vi "Teleop.vi"(10 "Match Info":T1={"Autonomous Elapsed Seconds"=0.0, "TeleOp Elapsed Seconds"=0.0, "Disabled Elapsed Seconds"=0.0, "Visited Autonomous"=FALSE, "Visited TeleOp"=FALSE, "Visited Disabled"=FALSE, "Autonomous Settings"={"Autonomous Style"=enum."Independent", "VI Refnum"=refnum}}, 11 "Call Context":T2) -> ()   [LabVIEW 2019]
doc: "This VI is called for each TeleOp packet received from the DS where the robot is not disabled. It is often used to read from the joysticks and update I/O or to update setpoints for timed control loops. It should complete and return within 20 milliseconds or it may miss DS packets."
uses:
  <vilib>/Rock Robotics/WPI/DriverStation/WPI_DriverStationDerivedRobotMode.ctl
  <vilib>/Rock Robotics/WPI/DriverStation/WPI_DriverStationMatch Info.ctl
  <vilib>/Rock Robotics/WPI/Solenoid/WPI_SolenoidValue.ctl
  <vilib>/Rock Robotics/WPI/Utilities/WPI_GetSetVariantRefNum.vi
  <vilib>/Rock Robotics/Network Tables/NT Write Boolean Array.vi
  <vilib>/Rock Robotics/Network Tables/NT Write Numeric Array.vi
  <vilib>/Rock Robotics/Network Tables/NT Read Boolean.vi
  <vilib>/Rock Robotics/Network Tables/NT Read Number.vi
  <vilib>/Rock Robotics/WPI/Solenoid/WPI_SolenoidSetEnum.vi
panel:
  in  "Auto speed switch":dbl=0.75
  out "Buttons":bool[](array[boolean])
  out "Axes":dbl[](array[numeric])
  out "Sample Slider 0":dbl(slide) scale=0.0..5.0
  out "Sample Boolean 1":bool
  # "REMEMBER BETWEEN 0 AND 1"
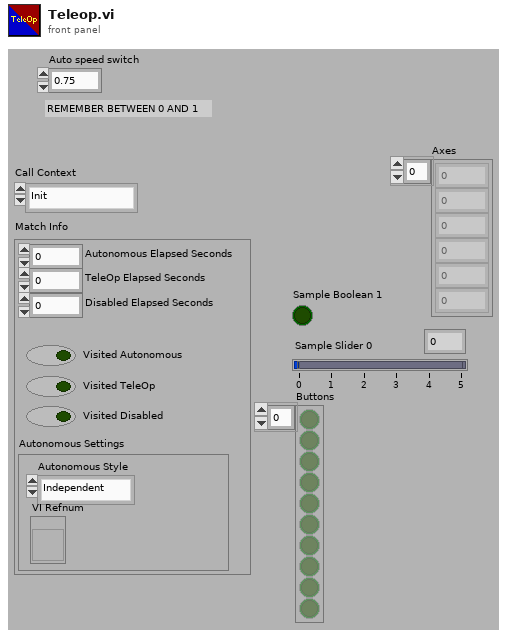
[diagram p1: front panel]
types:
  T1 = typedef "WPI_DriverStationMatch Info.ctl" = cluster{"Autonomous Elapsed Seconds":dbl, "TeleOp Elapsed Seconds":dbl, "Disabled Elapsed Seconds":dbl, "Visited Autonomous":bool, "Visited TeleOp":bool, "Visited Disabled":bool, "Autonomous Settings":cluster{"Autonomous Style":enum16{"Iterative", "Independent"}, "VI Refnum":refnum<vi>}}
  T2 = typedef "WPI_DriverStationDerivedRobotMode.ctl" = enum16{"Init", "Execute", "Stop"}
  T3 = typedef "WPI_JoystickDevRef.ctl" = cluster{"Device":T4}
  T4 = typedef "WPI_JoystickDeviceEnum.ctl" = enum16{"USB 0", "USB 1", "USB 2", "USB 3", "USB 4", "USB 5"}
  T5 = typedef "WPI_SolenoidValue.ctl" = enum16{"Off", "On", "Forward", "Reverse"}
  T6 = typedef "WPI_SolenoidDevRef.ctl" = cluster{"DevStatus":errorcluster, "Pneumatics Control Module":u8, "Forward Solenoid Channel":T7, "Reverse Solenoid Channel":T7}
  T7 = typedef "WPI_SolenoidChannel.ctl" = enum8{"Solenoid 0", "Solenoid 1", "Solenoid 2", "Solenoid 3", "Solenoid 4", "Solenoid 5", "Solenoid 6", "Solenoid 7", "Invalid"}
  T8 = typedef "WPI_RobotDriveDevRef.ctl" = cluster{"DevStatus":errorcluster, "Motors[]":T9[], "Square Inputs":bool, "Max Output":dbl}
  T9 = typedef "WPI_MotorControlDeviceRef.ctl" = cluster{"DeviceStatus":errorcluster, "Type":T10, "PWM":cluster{"PWM Channel":T11, "DeadBand":T12}, "CAN":cluster{"Device Number":u8, "SetOutput VI Ref":variant, "GetOutput VI Ref":variant, "Enable VI Ref":variant, "Disable VI Ref":variant, "Data":variant}, "Invert":bool, "DIO PWM":cluster{"PWM \"Enable\" Channel":T11, "DIOChannel":T13, "PWM Rate":dbl}}
  T10 = typedef "WPI_MotorControlType.ctl" = enum16{"PWM", "CAN", "DIO PWM"}
  T11 = typedef "FPGA_DIOPWMChannel.ctl" = enum8{"PWM 0", "PWM 1", "PWM 2", "PWM 3", "PWM 4", "PWM 5", "PWM 6", "PWM 7", "PWM 8", "PWM 9", "PWM MXP 0", "PWM MXP 1", "PWM MXP 2", "PWM MXP 3", "PWM MXP 4", "PWM MXP 5", "PWM MXP 6", "PWM MXP 7", "PWM MXP 8", "PWM MXP 9", "Invalid"}
  T12 = typedef "WPI_PWMDeadband.ctl" = cluster{"Name":string, "maxPositivePwm":i32, "minPositivePwm":i32, "centerPwm":i32, "maxNegativePwm":i32, "minNegativePwm":i32, "angularRange":u16}
  T13 = typedef "FPGA_DIOChannel.ctl" = enum8{"DIO 0", "DIO 1", "DIO 2", "DIO 3", "DIO 4", "DIO 5", "DIO 6", "DIO 7", "DIO 8", "DIO 9", "DIO MXP 0", "DIO MXP 1", "DIO MXP 2", "DIO MXP 3", "DIO MXP 4", "DIO MXP 5", "DIO MXP 6", "DIO MXP 7", "DIO MXP 8", "DIO MXP 9", "DIO MXP 10", "DIO MXP 11", "DIO MXP 12", "DIO MXP 13", "DIO MXP 14", "DIO MXP 15", "SPI Port CS1", "SPI Port CS2", "SPI Port CS3", "SPI Port MISO", "SPI Port MOSI", "Invalid"}
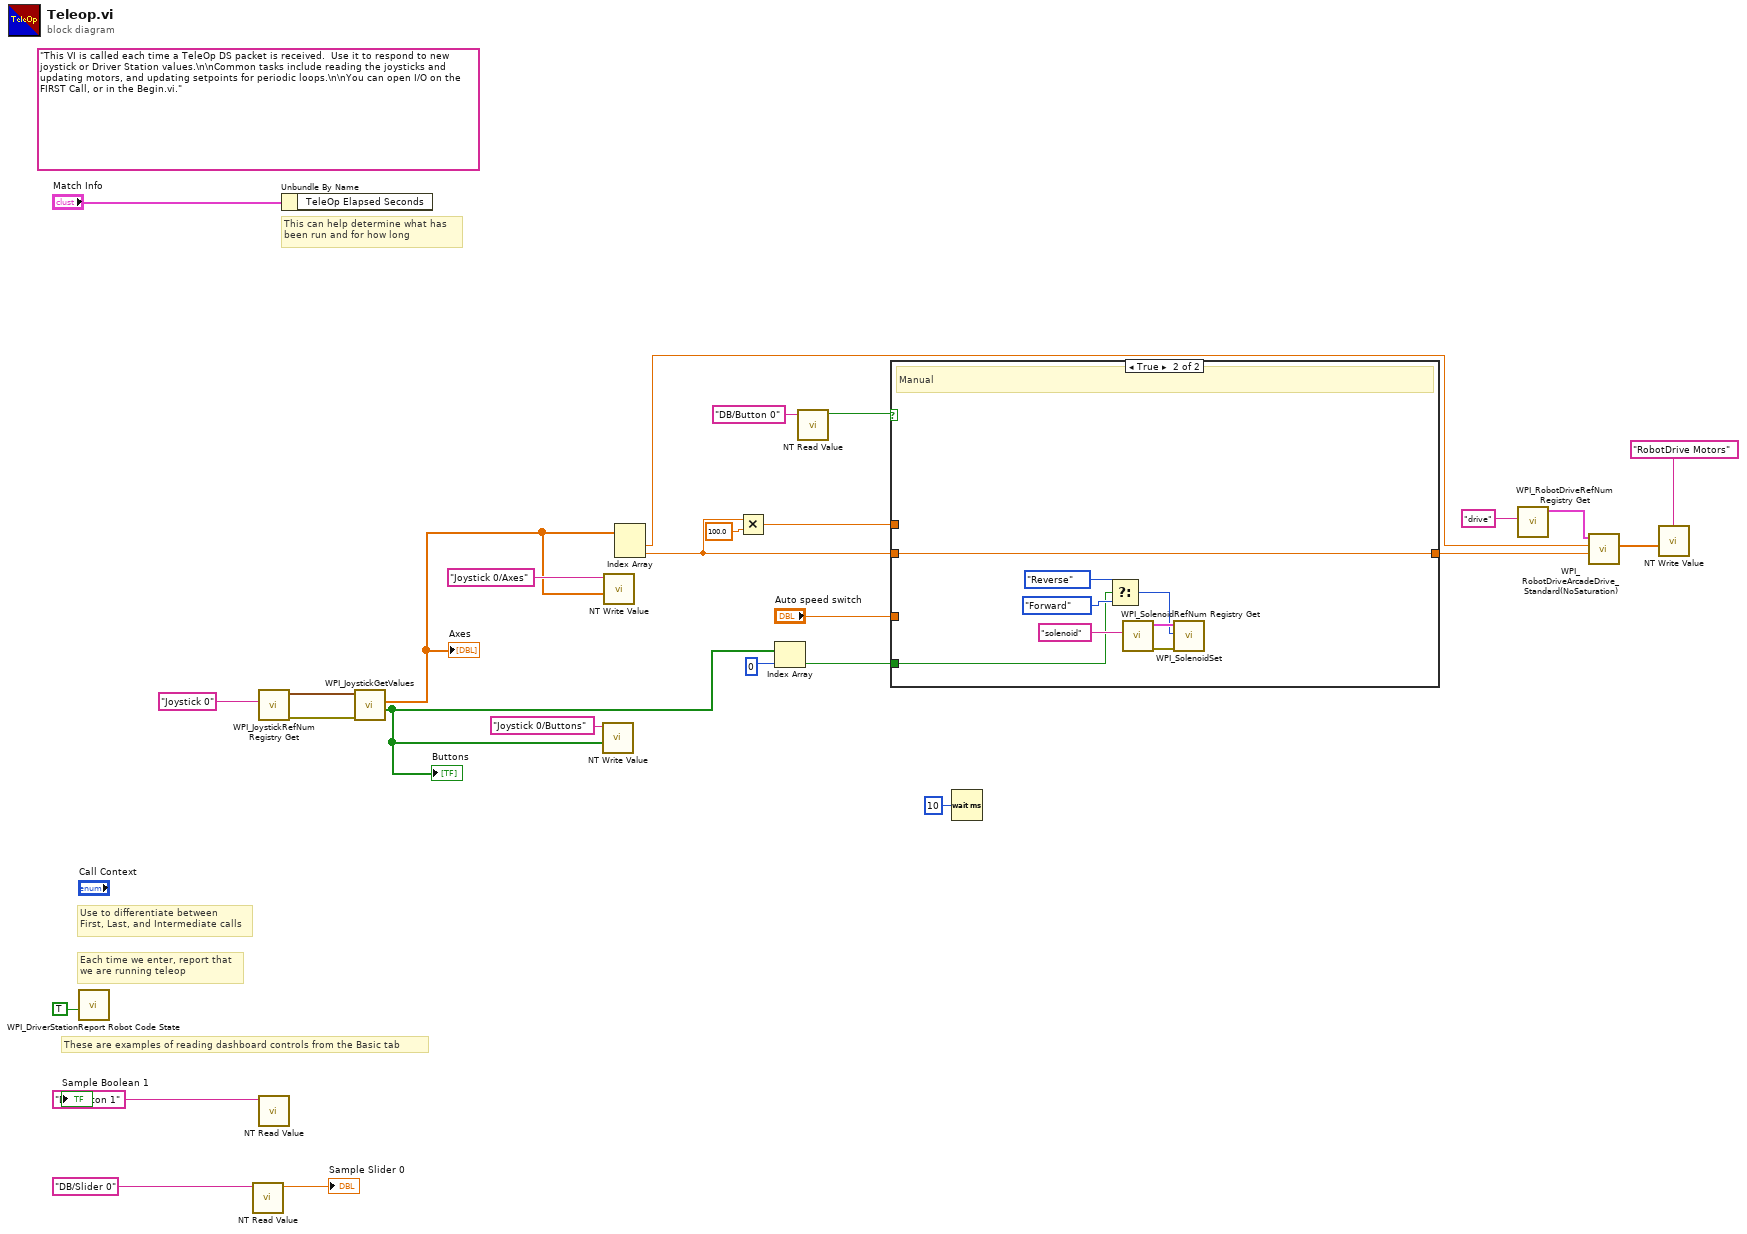
[diagram p0: block diagram]
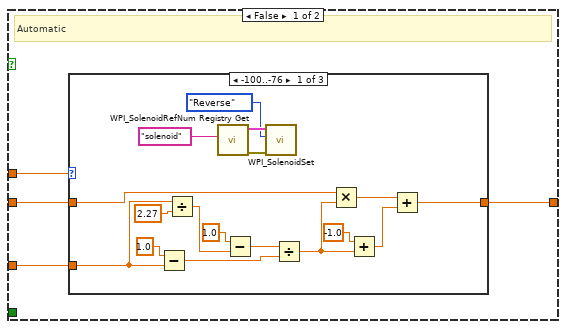
[diagram p2: hidden frame]
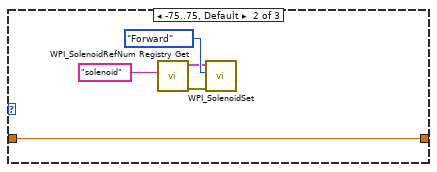
[diagram p3: hidden frame]
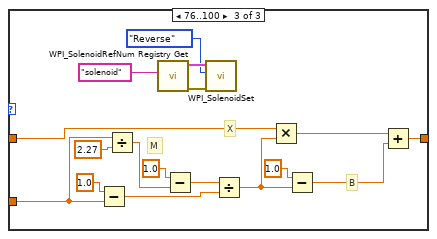
[diagram p4: hidden frame]
diagram:
  (unwired) "This VI is called each time a TeleOp DS packet is received.  Use it to respond to new joystick or Driver Station values.\n\nCommon tasks include reading the joysticks and updating motors, and updating setpoints for periodic loops.\n\nYou can open I/O on the FIRST Call, or in the Begin.vi."
  # "These are examples of reading dashboard controls from the Basic tab"
  # "Each time we enter, report that\nwe are running teleop"
  # "Use to differentiate between\nFirst, Last, and Intermediate calls"
  # "This can help determine what has\nbeen run and for how long"
  n1 = call <vilib>:"WPI_DriverStationReport Robot Code State.vi"("TeleOp"=TRUE ("Autonomous")) -> ()  [unwired: 10 in, 1 out]
  n2 = call-poly <vilib>:"NT Read Value.vi"("Name"="DB/Slider 0" ("refnum name")) -> ("Numeric"=→"Sample Slider 0":dbl)  [unwired: 9 in, 1 out]
  n3 = call <vilib>:"WPI_JoystickRefNum Registry Get.vi"("refnum name"="Joystick 0") -> ("error out"=w13:errorcluster, "JoystickDevRef"=w24:T3)  [unwired: 1 in, 8 out]
  n4 = call-poly <vilib>:"NT Read Value.vi"("Name"="DB/Button 1" ("refnum name")) -> ("Boolean"=→"Sample Boolean 1":bool)  [unwired: 9 in, 1 out]
  n5 = Unbundle By Name("Match Info") -> ()  [unwired: 1 out]
  n6 = call <vilib>:"WPI_JoystickGetValues.vi"("error in (no error)"=w13, "JoystickDevRef"=w24) -> ("Buttons"=w8:bool[], "Axes"=w20:dbl[])  [unwired: 5 in, 3 out]
  "Axes" <- w20
  "Buttons" <- w8
  n7 = call-poly <vilib>:"NT Write Value.vi"("Boolean Array"=w8, "Name"="Joystick 0/Buttons") -> ()  [unwired: 9 in, 1 out]
  n8 = call-poly <vilib>:"NT Write Value.vi"("Numeric Array"=w20, "Name"="Joystick 0/Axes") -> ()  [unwired: 9 in, 1 out]
  n9 = Index Array(array=w20) -> (element #1=w2:dbl, element #2=w7:dbl)  [unwired: 2 in]
  n10 = Multiply(x=w7, y=100.0) -> (x*y=w4:dbl)
  n11 = Index Array(array=w8, index=0) -> (element=w3:bool)
  n12 = call-poly <vilib>:"NT Read Value.vi"("Name"="DB/Button 0") -> ("Boolean"=w10:bool)  [unwired: 9 in, 1 out]
  n13 = case shown="True" w10 {
    tunnel: w4 -> [w32 _]
    tunnel: [w31 w79] -> w9
    tunnel: w7 -> [w30 w79]
    tunnel: "Auto speed switch" -> [w29 _]
    tunnel: w3 -> [_ w73]
    frame False {
      # "Automatic"
      n14 = case shown="-100..-76" w32 {
        tunnel: [w37 w50 w60] -> w31
        tunnel: w30 -> [w36 w50 w59]
        tunnel: w29 -> [w39 _ w61]
        frame -100..-76 {
          n15 = Subtract(x=1.0, y=w39) -> (x-y=w41:dbl)
          n16 = Divide(x=w39, y=2.27) -> (x/y=w38:dbl)
          n17 = call <vilib>:"WPI_SolenoidRefNum Registry Get.vi"("refnum name"="solenoid") -> ("error out"=w46:errorcluster, "SolenoidDevRef"=w48:T6)  [unwired: 9 in]
          n18 = Subtract(x=1.0, y=w38) -> (x-y=w43:dbl)
          n19 = call-poly <vilib>:"WPI_SolenoidSet.vi"("error in (no error)"=w46, "Value"=WPI_SolenoidValue."Reverse", "SolenoidDevRef"=w48) -> ()  [unwired: 7 in, 2 out]
          n20 = Divide(x=w43, y=w41) -> (x/y=w34:dbl)
          n21 = Multiply(x=w36, y=w34) -> (x*y=w40:dbl)
          n22 = Add(x=-1.0, y=w34) -> (x+y=w33:dbl)
          n23 = Add(x=w40, y=w33) -> (x+y=w37:dbl)
        }
        frame -75..75, Default {
          n24 = call <vilib>:"WPI_SolenoidRefNum Registry Get.vi"("refnum name"="solenoid") -> ("error out"=w51:errorcluster, "SolenoidDevRef"=w52:T6)  [unwired: 9 in]
          n25 = call-poly <vilib>:"WPI_SolenoidSet.vi"("error in (no error)"=w51, "Value"=WPI_SolenoidValue."Forward", "SolenoidDevRef"=w52) -> ()  [unwired: 7 in, 2 out]
        }
        frame 76..100 {
          # "B"
          # "M"
          # "X"
          n26 = Subtract(x=1.0, y=w61) -> (x-y=w63:dbl)
          n27 = Divide(x=w61, y=2.27) -> (x/y=w58:dbl)
          n28 = call <vilib>:"WPI_SolenoidRefNum Registry Get.vi"("refnum name"="solenoid") -> ("error out"=w68:errorcluster, "SolenoidDevRef"=w70:T6)  [unwired: 9 in]
          n29 = Subtract(x=1.0, y=w58) -> (x-y=w65:dbl)
          n30 = call-poly <vilib>:"WPI_SolenoidSet.vi"("error in (no error)"=w68, "Value"=WPI_SolenoidValue."Reverse", "SolenoidDevRef"=w70) -> ()  [unwired: 7 in, 2 out]
          n31 = Divide(x=w65, y=w63) -> (x/y=w56:dbl)
          n32 = Multiply(x=w59, y=w56) -> (x*y=w62:dbl)
          n33 = Subtract(x=1.0, y=w56) -> (x-y=w55:dbl)
          n34 = Add(x=w62, y=w55) -> (x+y=w60:dbl)
        }
      }
    }
    frame True {
      # "Manual"
      n35 = Select(t=WPI_SolenoidValue."Reverse" ("Value"), s=w73, f=WPI_SolenoidValue."Forward") -> (s? t:f=w77:T5)
      n36 = call <vilib>:"WPI_SolenoidRefNum Registry Get.vi"("refnum name"="solenoid") -> ("error out"=w76:errorcluster, "SolenoidDevRef"=w78:T6)  [unwired: 9 in]
      n37 = call-poly <vilib>:"WPI_SolenoidSet.vi"("error in (no error)"=w76, "Value"=w77, "SolenoidDevRef"=w78) -> ()  [unwired: 7 in, 2 out]
    }
  }
  n38 = Wait (ms)(milliseconds to wait=u32 10) -> ()  [unwired: 1 out]
  n39 = call <vilib>:"WPI_RobotDriveRefNum Registry Get.vi"("refnum name"="drive") -> ("RobotDriveDevRef"=w26:T8)  [unwired: 1 in, 9 out]
  n40 = call <vilib>:"WPI_RobotDriveArcadeDrive_Standard(NoSaturation).vi"("Y axis value"=w9, "X axis value"=w2, "RobotDriveDevRef"=w26) -> ("Motor Values"=w15:dbl[])  [unwired: 1 in, 7 out]
  n41 = call-poly <vilib>:"NT Write Value.vi"("Numeric Array"=w15, "Name"="RobotDrive Motors") -> ()  [unwired: 9 in, 1 out]
